vi "getEndRampEvent.vi"(8 "error in (no error)":errorcluster, 11 "RampAction in":refnum<class "RampAction.lvclass">) -> (0 "error out":errorcluster, 2 "EndScriptEvent":refnum<class "ScriptEvent.lvclass">, 3 "RampAction out":refnum<class "RampAction.lvclass">)   [LabVIEW 2009, in "Views.lvlib" / "ScriptEditor.lvlib" / "RampAction.lvclass"]
uses:
  RampAction.lvclass
  Tools/Scripting/ScriptingEvent/ScriptEvent.lvclass
  Tools/Scripting/ScriptingEvent/ScriptEvents/Ramp/RampEvent/RampEvent.lvclass
  ActionPanel.lvclass
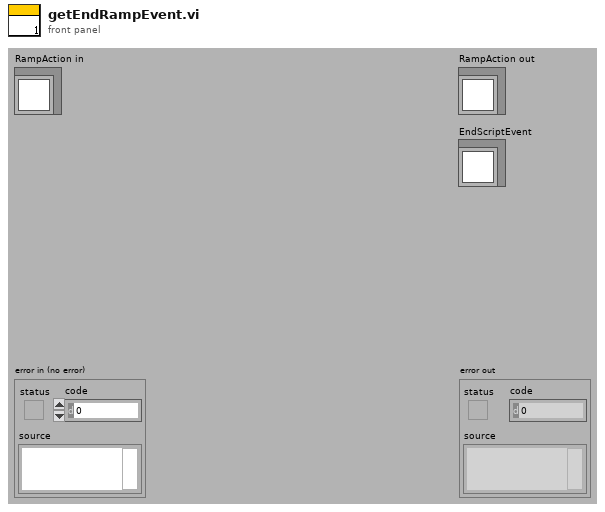
[diagram p1: front panel]
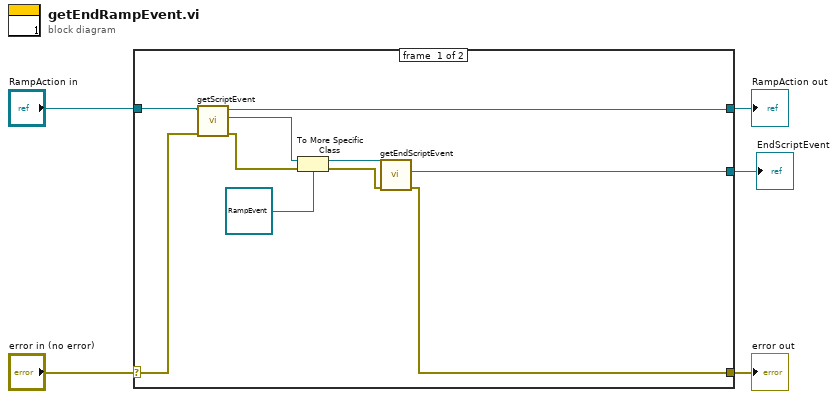
[diagram p0: block diagram]
diagram:
  n1 = case shown="No Error" "error in (no error)" {
    selector: "error in (no error)" -> [w7 w17]
    tunnel: [w8 w17] -> w4
    tunnel: [w14 w16] -> w2
    tunnel: "RampAction in" -> [w15 w16]
    tunnel: [w10 _] -> w1
    frame #0 {
      n2 = call "getScriptEvent.vi"("error in (no error)"=w7, "ActionPanel.lvclass in"=w15) -> ("error out"=w6:errorcluster, "ScriptEvent.lvclass"=w13:refnum<class "ScriptEvent.lvclass">, "ActionPanel.lvclass out"=w14:refnum<class "RampAction.lvclass">)  [unwired: 7 in]
      n3 = To More Specific Class(target class=refnum<class "RampEvent.lvclass"> refnum ("Tools.lvlib:Scripting.lvlib:RampEvent.lvclass"), reference=w13, error in=w6) -> (specific class reference=w12:refnum<class "RampEvent.lvclass">, error out=w9:errorcluster)
      n4 = call "getEndScriptEvent.vi"("error in (no error)"=w9, "RampEvent.lvclass in"=w12) -> ("error out"=w8:errorcluster, "ScriptEvent.lvclass"=w10:refnum<class "ScriptEvent.lvclass">)  [unwired: 7 in, 1 out]
    }
    frame #1 {
    }
  }
  "error out" <- w4
  "RampAction out" <- w2
  "EndScriptEvent" <- w1
